vi "DebResetLog.vi"(5 "error in":errorcluster) -> (19 "error out":errorcluster)   [LabVIEW 2017]
uses:
  DebCommandLog.vi
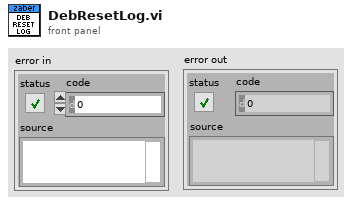
[diagram p1: front panel]
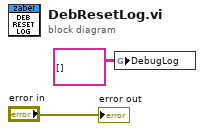
[diagram p0: block diagram]
diagram:
  n1 = global write "DebCommandLog.vi" "DebugLog"(string[][] [] ("DebugLog")) -> ()
  "error out" <- "error in"
